vi "ForceLoop.vi"(7 "Inputs":T2 {"Color Pane" items=["Blue", "Red", "Green", "Saturation", "Value", "Intensity", "Luminance", "Hue", ""]}, 8 "error in":errorcluster, 9 "Time":dbl format="%#_13g", 10 "Slope":dbl format="%#_13g", 11 "task/channels in":refnum<k21>) -> (0 "error out":errorcluster, 2 "Force Cluster":T1, 3 "task out":refnum<k21>, 4 "Time Exceeded?":bool)   [LabVIEW 2020]
uses:
  Inputs.ctl
  <vilib>/DAQmx/read.llb/DAQmx Read (Analog 1D DBL 1Chan NSamp).vi
  <vilib>/DAQmx/miscellaneous.llb/DAQmx Fill In Error Info.vi
  <vilib>/addons/control/pid/pid.llb/PID (DBL).vi
  <vilib>/Simulation/Implementation/XNodeFramework/SimXNode/SimX.xnode
  <vilib>/Simulation/Model Libraries/Controllers/SIM SISO Controller.vi
  <vilib>/Simulation/Model Libraries/Controllers/SIM Controller (Forward Path).vi
  <vilib>/addons/control/pid/NI_PID_pid.lvlib
  <vilib>/Simulation/Implementation/Shared/SIMSCR Execution Mode.ctl
  <vilib>/Simulation/Scripting/Companion Diagram/SimConfigNode/_simSolvers.ctl
  <vilib>/Simulation/Scripting/Companion Diagram/SimConfigNode/SimParams.ctl
  <vilib>/Simulation/Scripting/Companion Diagram/SimConfigNode/SimDog.xnode
  <vilib>/Simulation/Implementation/Shared/SIM Bundle Sim Info.vi
  <vilib>/Simulation/Implementation/Shared/SIM Unbundle Sim Info.vi
  <vilib>/Simulation/Implementation/Shared/NILVSim_FinalizeModel.vi
  <vilib>/Simulation/Implementation/Shared/NILVSim_GetModelError.vi
  <vilib>/Simulation/Implementation/Shared/NILVSim_Initialize.vi
  <vilib>/Simulation/Utility/Implementation/NILVSim Get Time and IsAcceptedStep.vi
  <vilib>/Simulation/Implementation/Shared/NILVSim_Manager.vi
  <vilib>/Simulation/Implementation/Shared/NI_SIM_Implementation.lvlib
  <vilib>/Simulation/Implementation/Shared/NILVSIM_BeginStep.vi
  <vilib>/Simulation/Param Hierarchy/Typedefs/SIMPH Param Control Actions.ctl
  <vilib>/Simulation/Implementation/Shared/NILVSim_ParamChanged.vi
  <vilib>/Utility/error.llb/Clear Errors.vi
  <vilib>/Simulation/Implementation/Shared/SIMSH Read Queue.vi
  <vilib>/addons/Control Design/_Model Construction/Model Typedefs.llb/CD Zero-Pole-Gain Model (SISO).ctl
  <vilib>/addons/Control Design/_Model Construction/NI_LinSys_Model Typedefs.lvlib
  <vilib>/addons/Control Design/_Model Construction/Model Typedefs.llb/CD General Elements.ctl
  <vilib>/addons/Control Design/_Model Construction/Model Typedefs.llb/CD Zero-Pole-Gain Model (MIMO).ctl
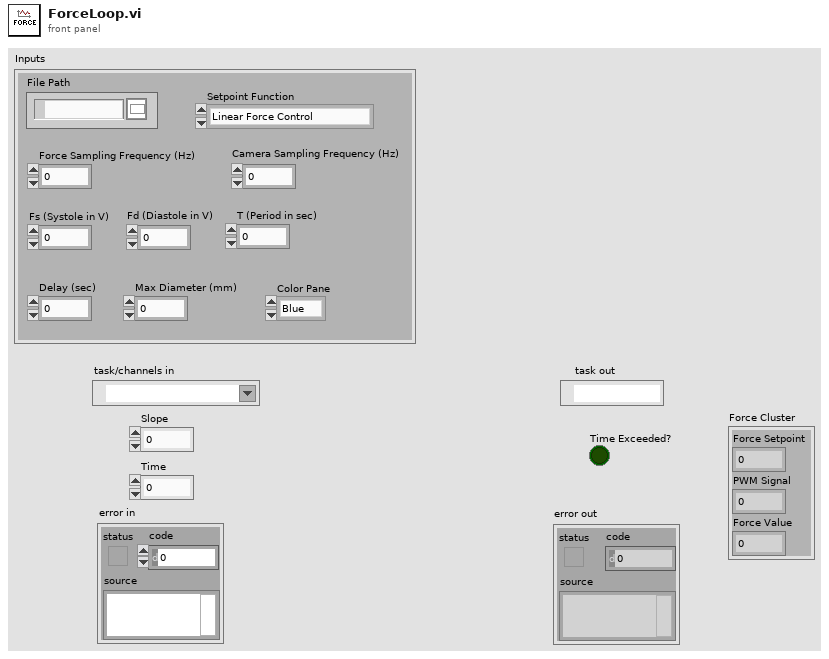
[diagram p1: front panel]
types:
  T1 = cluster{"Force Setpoint":dbl, "PWM Signal":dbl, "Force Value":dbl}
  T2 = typedef "Inputs.ctl" = cluster{"File Path":path, "Force Sampling Frequency (Hz)":dbl, "Camera Sampling Frequency (Hz)":dbl, "Fs (Systole in V)":dbl, "Fd (Diastole in V)":dbl, "T (Period in sec)":dbl, "Delay (sec)":dbl, "Setpoint Function":enum16{"Linear Force Control", "Sinusoidal Force Control", "Blood-Pressure Force Control"}, "Max Diameter (mm)":dbl, "Color Pane":i32}
  T3 = enum16{"Linear Force Control", "Sinusoidal Force Control", "Blood-Pressure Force Control"}
  T4 = enum16{"Simulate to Completion", "Single Time-Step Simulation (Fixed Step Only)"}
  T5 = typedef "SIMSCR Execution Mode.ctl" = enum16{"Simulate to Completion", "Single Time-Step Simulation (Fixed Step Only)"}
  T6 = typedef "SIMPH Param Control Actions.ctl" = enum16{"get params", "set params"}
  T7 = typedef "NI_LinSys_Model Typedefs.lvlib/CD Zero-Pole-Gain Model (MIMO).ctl" = cluster{"properties":T8, "zero-pole-gain(s)":T9[][]}
  T8 = typedef "NI_LinSys_Model Typedefs.lvlib/CD General Elements.ctl" = cluster{"Model name":string, "Input names":string[], "Output names":string[], "Input Delays":dbl[], "Output Delays":dbl[], "Sampling Time":dbl, "Notes":string}
  T9 = typedef "NI_LinSys_Model Typedefs.lvlib/CD Zero-Pole-Gain Model (SISO).ctl" = cluster{"Gain":dbl, "Zeros":cdb[], "Poles":cdb[], "delay":dbl}
  T10 = cluster{"SIMSH Sim Time":dbl, "Output Range":cluster{"output high":dbl, "output low":dbl}, "Unbundle By Name":cluster{"output high":dbl, "output low":dbl}, "Saturation":cluster{"output":dbl}, "Select":cluster{"s? t:f":dbl}, "Reciprocal":cluster{"1/x":dbl}, "Select 3":cluster{"s? t:f":dbl}, "Equal To 0?":cluster{"x = 0?":bool}, "Summation 3":cluster{"Result":dbl}, "Gain 2":cluster{"output":dbl}, "Summation 2":cluster{"Result":dbl}, "Zero-Pole-Gain":cluster{"output y(t)":dbl}, "cd_Check If System has Integrator (ZPK).vi":cluster{"Integrator?":bool}}
  T11 = typedef "SimParams.ctl" = cluster{"Initial Time (s)":dbl, "Final Time (s)":dbl, "Step Size (s)":dbl, "ODE Solver":T12, "Minimum Step Size (s)":dbl, "Maximum Step Size (s)":dbl, "Relative Tolerance":dbl, "Absolute Tolerance":dbl, "Software Timing":bool, "Initial Step Size (s)":dbl, "Automatic Fixed Step Size?":bool, "Automatic Discrete Step Size?":bool, "Discrete Step Size (s)":dbl, "Calculate using Time Step":bool, "Solver Wired?":bool, "Prev.Frm.Expected End":u64, "Prev.Frm.Actual End":u64, "Prev.Frm.Finished Late?":bool, "Prev.Iter.Expected End":u64, "Prev.Iter.Actual End":u64, "Prev.Iter.Finished Late?":bool, "Expected Iteration Start":u64, "Actual Iteration Start":u64, "Expected Frame Start":u64, "Actual Frame Start":u64, "Source Name":string, "Name":string, "Period":i64, "Deadline":i64, "Offset":i64, "Start":i64, "Priority":i32, "Timeout":i32, "Processor":i32, "Mode":enum32{"No Change", "Process missed periods, maintain original phase", "Discard missed periods, maintain original phase", "Process missed periods, ignore original phase", "Discard missed periods, ignore original phase"}, "Wakeup reason":enum32{"Normal", "Aborted", "Asynchronous wakeup", "Timing source error", "Timed loop error", "Timeout"}, "Error":errorcluster, "Source Type":string, "Secondary Source Type":string, "Global End Time":u64, "Global Start Time":u64, "Full Solver Reset":bool, "Execution Mode":T5, "Nan/Inf Check":bool, "Custom Solver Library":string, "Solver Is Variable":bool, "custom solver name":string, "Signal Collection Decimation":u32}
  T12 = typedef "_simSolvers.ctl" = enum16{"Runge-Kutta 1 (Euler)", "Runge-Kutta 2", "Runge-Kutta 3", "Runge-Kutta 4", "Runge-Kutta 23 (variable)", "Runge-Kutta 45 (variable)", "BDF (variable)", "Adams-Moulton (variable)", "Rosenbrock (variable)", "Discrete States Only", "SDIRK 4 (variable)", "Radau 5 (variable)", "Radau 9 (variable)", "Radau 13 (variable)", "Radau [Variable Order] (variable)", "Gear's Method (variable)", "Linearizer", "State Query", "Trim Eval", "Custom Solver"}
  T13 = cluster{"proportional gain (Kc)":dbl, "integral time (Ti, min)":dbl, "derivative time (Td, min)":dbl}
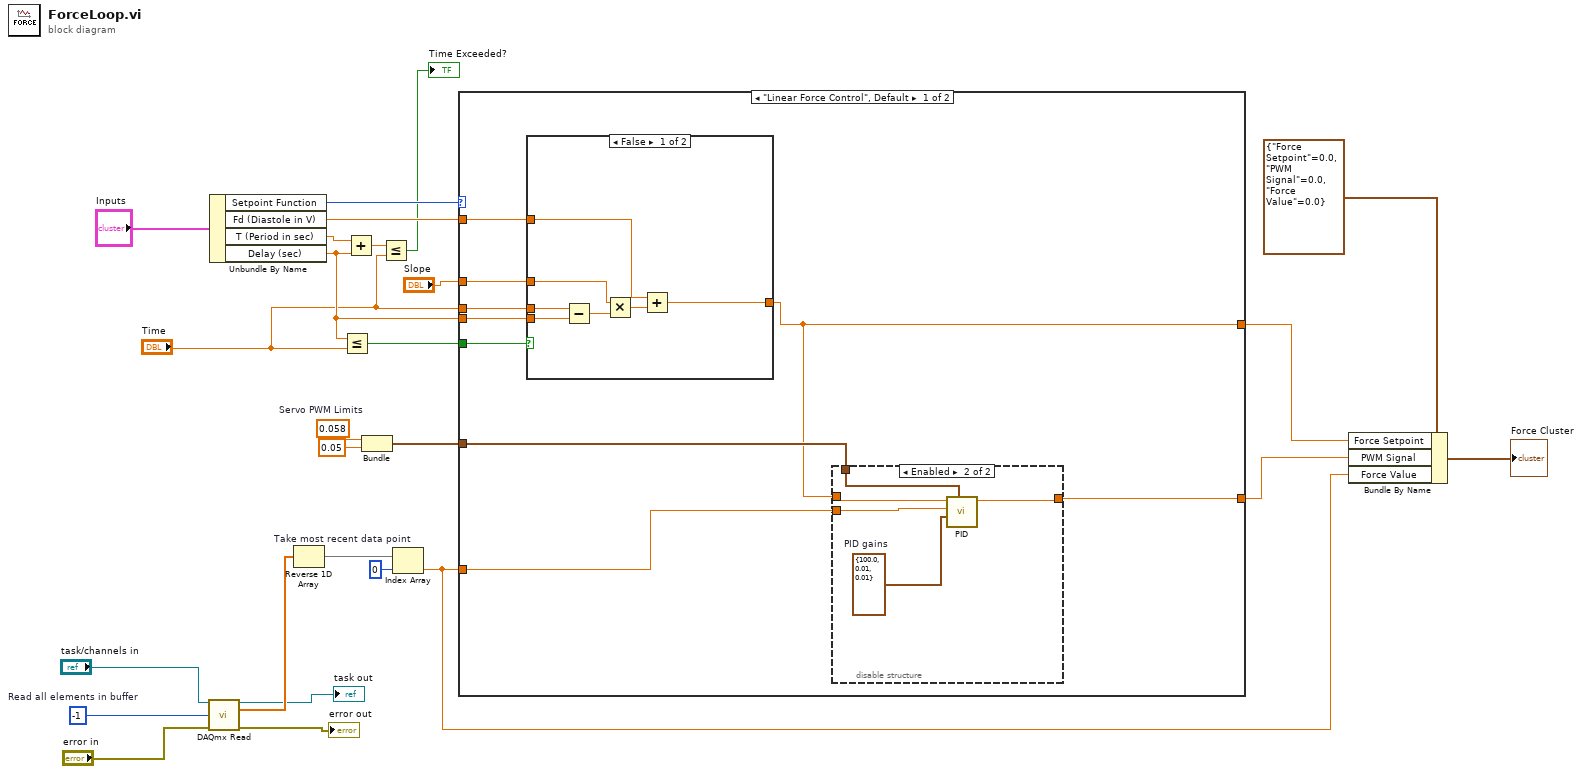
[diagram p0: block diagram]
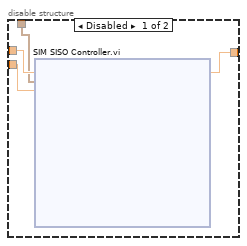
[diagram p2: hidden frame]
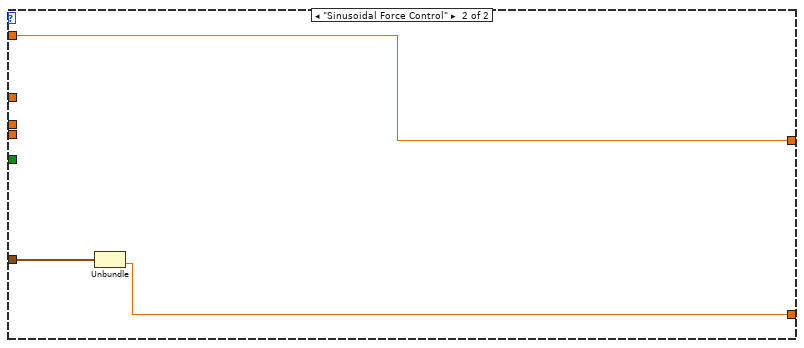
[diagram p4: hidden frame]
diagram:
  w14 = -1  # Read all elements in buffer
  w22 = 0.058  # Servo PWM Limits
  n1 = call-poly <vilib>:"DAQmx Read.vi"("task/channels in"="task/channels in", "number of samples per channel"=w14, "error in"="error in") -> ("task out"=→"task out":refnum<k21>, "data"=w13:dbl[], "error out"=→"error out":errorcluster)  [unwired: 10 in]
  n2 = Unbundle By Name("Inputs") -> ("Setpoint Function"=w25:T3, "Fd (Diastole in V)"=w18:dbl, "T (Period in sec)"=w23:dbl, "Delay (sec)"=w20:dbl)
  n3 = Reverse 1D Array(array=w13) -> (reversed array=w12:dbl[])
  n4 = Less Or Equal?(x=w20, y="Time") -> (x <= y?=w21:bool)
  n5 = Add(x=w23, y=w20) -> (x+y=w17:dbl)
  n6 = Bundle("Servo PWM Limits"=w22, 0.05) -> (w8:cluster{"Servo PWM Limits":dbl, dbl})  [unwired: 1 in]
  n7 = Less Or Equal?(x=w17, y="Time") -> (x <= y?=→"Time Exceeded?":bool)
  n8 = Index Array "Take most recent data point"(array=w12, index=0) -> (element=w4:dbl)
  n9 = case shown="\"Linear Force Control\", Default" w25 {
    tunnel: w21 -> [w35 _]
    tunnel: w20 -> [w34 _]
    tunnel: "Time" -> [w33 _]
    tunnel: "Slope" -> [w32 _]
    tunnel: w18 -> [w31 w327]
    tunnel: w8 -> [w30 w326]
    tunnel: w4 -> [w29 _]
    tunnel: [w28 w325] -> w5
    tunnel: [w27 w327] -> w6
    frame "Linear Force Control", Default {
      n10 = case shown="False" w35 {
        tunnel: w34 -> [w323 _]
        tunnel: w33 -> [w322 _]
        tunnel: w32 -> [w318 _]
        tunnel: w31 -> [w320 w324]
        tunnel: [w317 w324] -> w27
        frame False {
          n11 = Subtract(x=w322, y=w323) -> (x-y=w319:dbl)
          n12 = Multiply(x=w318, y=w319) -> (x*y=w321:dbl)
          n13 = Add(x=w320, y=w321) -> (x+y=w317:dbl)
        }
        frame True {
        }
      }
      n14 = disable-structure shown="Enabled" {
        disable-tunnel: [w39 w316] -> w28
        disable-tunnel: w27 -> [w38 w315]
        disable-tunnel: w30 -> [w36 w314]
        disable-tunnel: w29 -> [w37 w313]
        frame Disabled {
          n15 = xnode "SIM SISO Controller.vi"("Setpoint"=w38, "Output Range"=w36, "Measurement"=w37) -> ("Output"=w39:dbl)  [unwired: 3 in, 6 out]
        }
        frame Enabled {
          w312 = T13 {"proportional gain (Kc)"=100.0, "integral time (Ti, min)"=0.01, "derivative time (Td, min)"=0.01}  # PID gains
          n16 = call-poly <vilib>:"PID.vi"("output range"=w314, "PID gains"=w312, "process variable"=w313, "setpoint"=w315) -> ("output"=w316:dbl)  [unwired: 6 in, 1 out]
        }
      }
    }
    frame "Sinusoidal Force Control" {
      n17 = Unbundle(w326) -> (w325:dbl)  [unwired: 1 out]
    }
  }
  n18 = Bundle By Name(cluster=T1 {"Force Setpoint"=0.0, "PWM Signal"=0.0, "Force Value"=0.0}, "Force Setpoint"=w6, "PWM Signal"=w5, "Force Value"=w4) -> (→"Force Cluster":T1)
